vi "Initialize_COM_Port.vi"(8 "error out":errorcluster caption="error in", 11 "VISA resource name IN":refnum<visa-resource-name>="COM3") -> (0 "error out 2":errorcluster caption="error out", 3 "VISA resource name OUT":refnum<visa-resource-name>, 4 "COM ok":bool)   [LabVIEW 2017]
uses:
  <vilib>/Instr/_visa.llb/VISA Set IO Buffer Mask.ctl
panel:
  in  "Cancel":bool
  # "Action in Progress"
  # "1. Initialization of COM - Port Parameters\n\n2. Establish serial Connection to the IMU Board"
  # "Status"
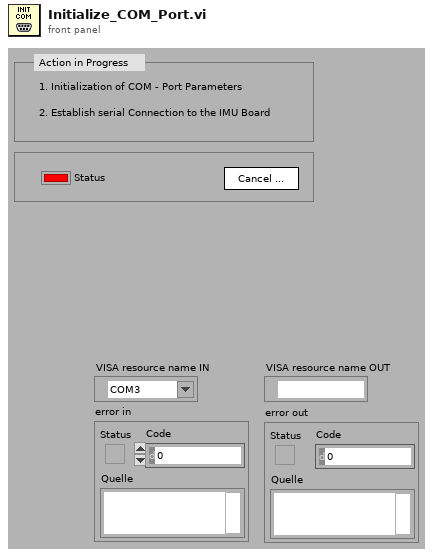
[diagram p1: front panel]
types:
  T1 = typedef "VISA Set IO Buffer Mask.ctl" = u16
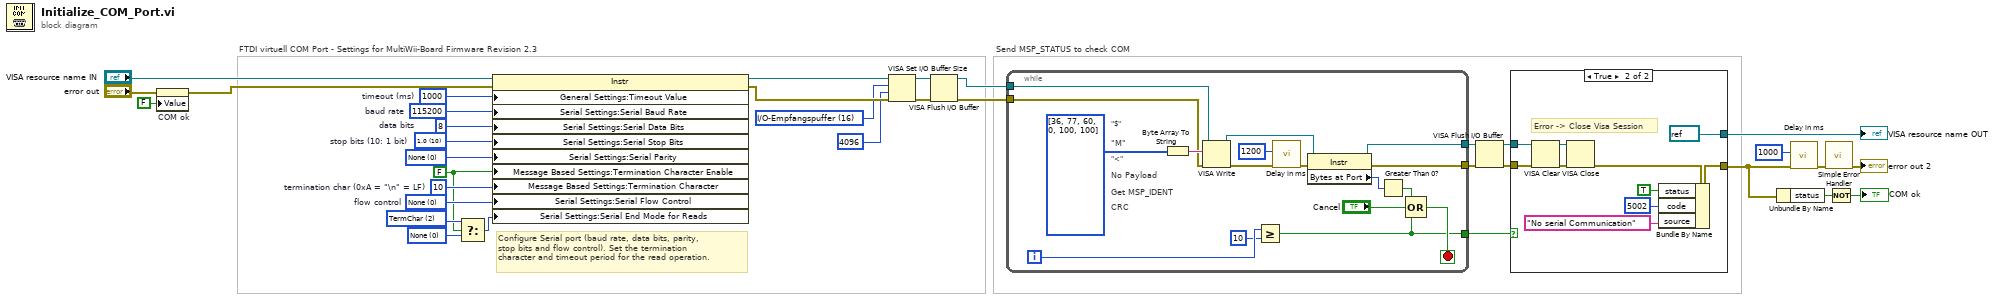
[diagram p0: block diagram]
diagram:
  w16 = u16 0 items=["None", "Odd", "Even", "Mark", "Space"] ("Serial Settings:Parity")
  w19 = T1 16 items=["I/O-Empfangspuffer"=16, "I/O-Übertragungspuffer"=32, "I/O-Empfangs- und Übertragungspuffer"=48] ("Mask")
  w26 = FALSE ("End read on termination character?")
  w29 = u16 0 items=["None"=0, "XON/XOFF"=1, "RTS/CTS"=2, "DTR/DSR"=4]  # flow control
  w30 = u8 10  # termination char (0xA = "\n" = LF)
  w31 = u16 10 items=["1.0"=10, "1.5"=15, "2.0"=20]  # stop bits (10: 1 bit)
  w32 = u16 8  # data bits
  w33 = u32 115200  # baud rate
  w34 = u32 1000  # timeout (ms)
  w27 = u16 0 items=["None", "LastBit", "TermChar"] ("Serial Settings:Serial End Mode for Reads")
  w28 = u16 2 items=["None", "LastBit", "TermChar"] ("Serial Settings:Serial End Mode for Reads")
  # "Send MSP_STATUS to check COM"
  # "FTDI virtuell COM Port - Settings for MultiWii-Board Firmware Revision 2.3"
  # "Configure Serial port (baud rate, data bits, parity,\nstop bits and flow control). Set the termination\ncharacter and timeout period for the read operation."
  n1 = property on="COM ok" class="Bool (strict)"(error in="error out", "Value"=FALSE ("COM ok")) -> (error out=w4:errorcluster)  [unwired: 1 in, 1 out]
  n2 = Select(t=w28, s=w26, f=w27) -> (s? t:f=w25:u16)
  n3 = property class="Instr"(reference="VISA resource name IN", error in=w4, "General Settings:Timeout Value"=w34, "Serial Settings:Serial Baud Rate"=w33, "Serial Settings:Serial Data Bits"=w32, "Serial Settings:Serial Stop Bits"=w31, "Serial Settings:Serial Parity"=w16, "Message Based Settings:Termination Character Enable"=w26, "Message Based Settings:Termination Character"=w30, "Serial Settings:Serial Flow Control"=w29, "Serial Settings:Serial End Mode for Reads"=w25) -> (reference out=w22:refnum<visa-resource-name>, error out=w21:errorcluster)
  n4 = VISA Set I/O Buffer Size(VISA resource name=w22, mask (16)=w19, size (4096)=u32 4096 ("Größe (4096)"), error in (no error)=w21) -> (VISA resource name out=w17:refnum<visa-resource-name>, error out=w18:errorcluster)
  n5 = VISA Flush I/O Buffer(VISA resource name=w17, error in (no error)=w18) -> (VISA resource name out=w1:refnum<visa-resource-name>, error out=w2:errorcluster)  [unwired: 1 in]
  n6 = while {
    tunnel: w1 -> [w52]
    tunnel: [w43] -> w15
    tunnel: [w44] -> w14
    tunnel: [w38] -> w13
    tunnel: w2 -> [w37]
    i -> [w48]
    stop <- w46 stop-if-true
    # "CRC"
    # "Get MSP_IDENT"
    # "No Payload"
    # "\"<\""
    # "\"M\""
    # "\"$\""
    n7 = Byte Array To String(unsigned byte array=u8[] [36, 77, 60, 0, 100, 100]) -> (string=w51:string)
    n8 = VISA Write(VISA resource name=w52, write buffer=w51, error in (no error)=w37) -> (VISA resource name out=w50:refnum<visa-resource-name>, error out=w42:errorcluster)  [unwired: 1 out]
    n9 = Greater Or Equal?(x=w48, y=10) -> (x >= y?=w38:bool)
    n10 = call "Delay in ms.vi"("error in (no error)"=w42, "Delay Time [ms]"=u32 1200 ("Delay (ms)")) -> ("error out"=w40:errorcluster)  [unwired: 9 in]
    n11 = property class="Instr"(reference=w50, error in=w40) -> (reference out=w43:refnum<visa-resource-name>, error out=w44:errorcluster, "Bytes at Port"=w49:u32)
    n12 = Greater Than 0?(x=w49) -> (x > 0?=w45:bool)
    n13 = Compound Arithmetic op=OR(w45, "Cancel", w38) -> (w46:bool)
  }
  n14 = VISA Flush I/O Buffer(VISA resource name=w15, error in (no error)=w14) -> (VISA resource name out=w11:refnum<visa-resource-name>, error out=w12:errorcluster)  [unwired: 1 in]
  n15 = case shown="True" w13 {
    tunnel: w12 -> [w54 w60]
    tunnel: w11 -> [w53 w56]
    tunnel: [w54 w61] -> w9
    tunnel: [w53 refnum<visa-resource-name> refnum ("VISA resource name OUT 2")] -> w10
    frame False {
    }
    frame True {
      # "Error -> Close Visa Session"
      n16 = VISA Clear(VISA resource name=w56, error in (no error)=w60) -> (VISA resource name out=w57:refnum<visa-resource-name>, error out=w59:errorcluster)
      n17 = VISA Close(VISA resource name=w57, error in (no error)=w59) -> (error out=w58:errorcluster)
      n18 = Bundle By Name(cluster=w58, "status"=TRUE, "code"=5002, "source"="No serial Communication") -> (w61:errorcluster)
    }
  }
  "VISA resource name OUT" <- w10
  n19 = Unbundle By Name(w9) -> ("status"=w24:bool)
  n20 = call "Delay in ms.vi"("error in (no error)"=w9, "Delay Time [ms]"=u32 1000) -> ("error out"=w7:errorcluster)  [unwired: 9 in]
  n21 = call <vilib>:"Simple Error Handler.vi"("error in (no error)"=w7) -> ("error out"=→"error out 2":errorcluster)  [unwired: 4 in, 4 out]
  n22 = Not(x=w24) -> (.not. x?=→"COM ok":bool)
